vi "Energy(B)INIT.vi"(7 "B [T] in":dbl=1.0, 10 "calib(pixel) out in":T7, 11 "Cam in":T1) -> (2 "calib(pixel) out out":T7, 3 "Cam out 2":T1)   [LabVIEW 2013]
uses:
  calibPixel.ctl
  CamSettingSUB_TypDEf.ctl
  MagAnalysis_Online_Bella/SubVis/CamAndObj_TypDEf.ctl
  shared/OnOffTypeDef.ctl
  userROI.ctl
  shared/numericVariable_TypeDef.ctl
  CamRoiTypDef.ctl
  BaseDriver/BaseDriver.lvclass
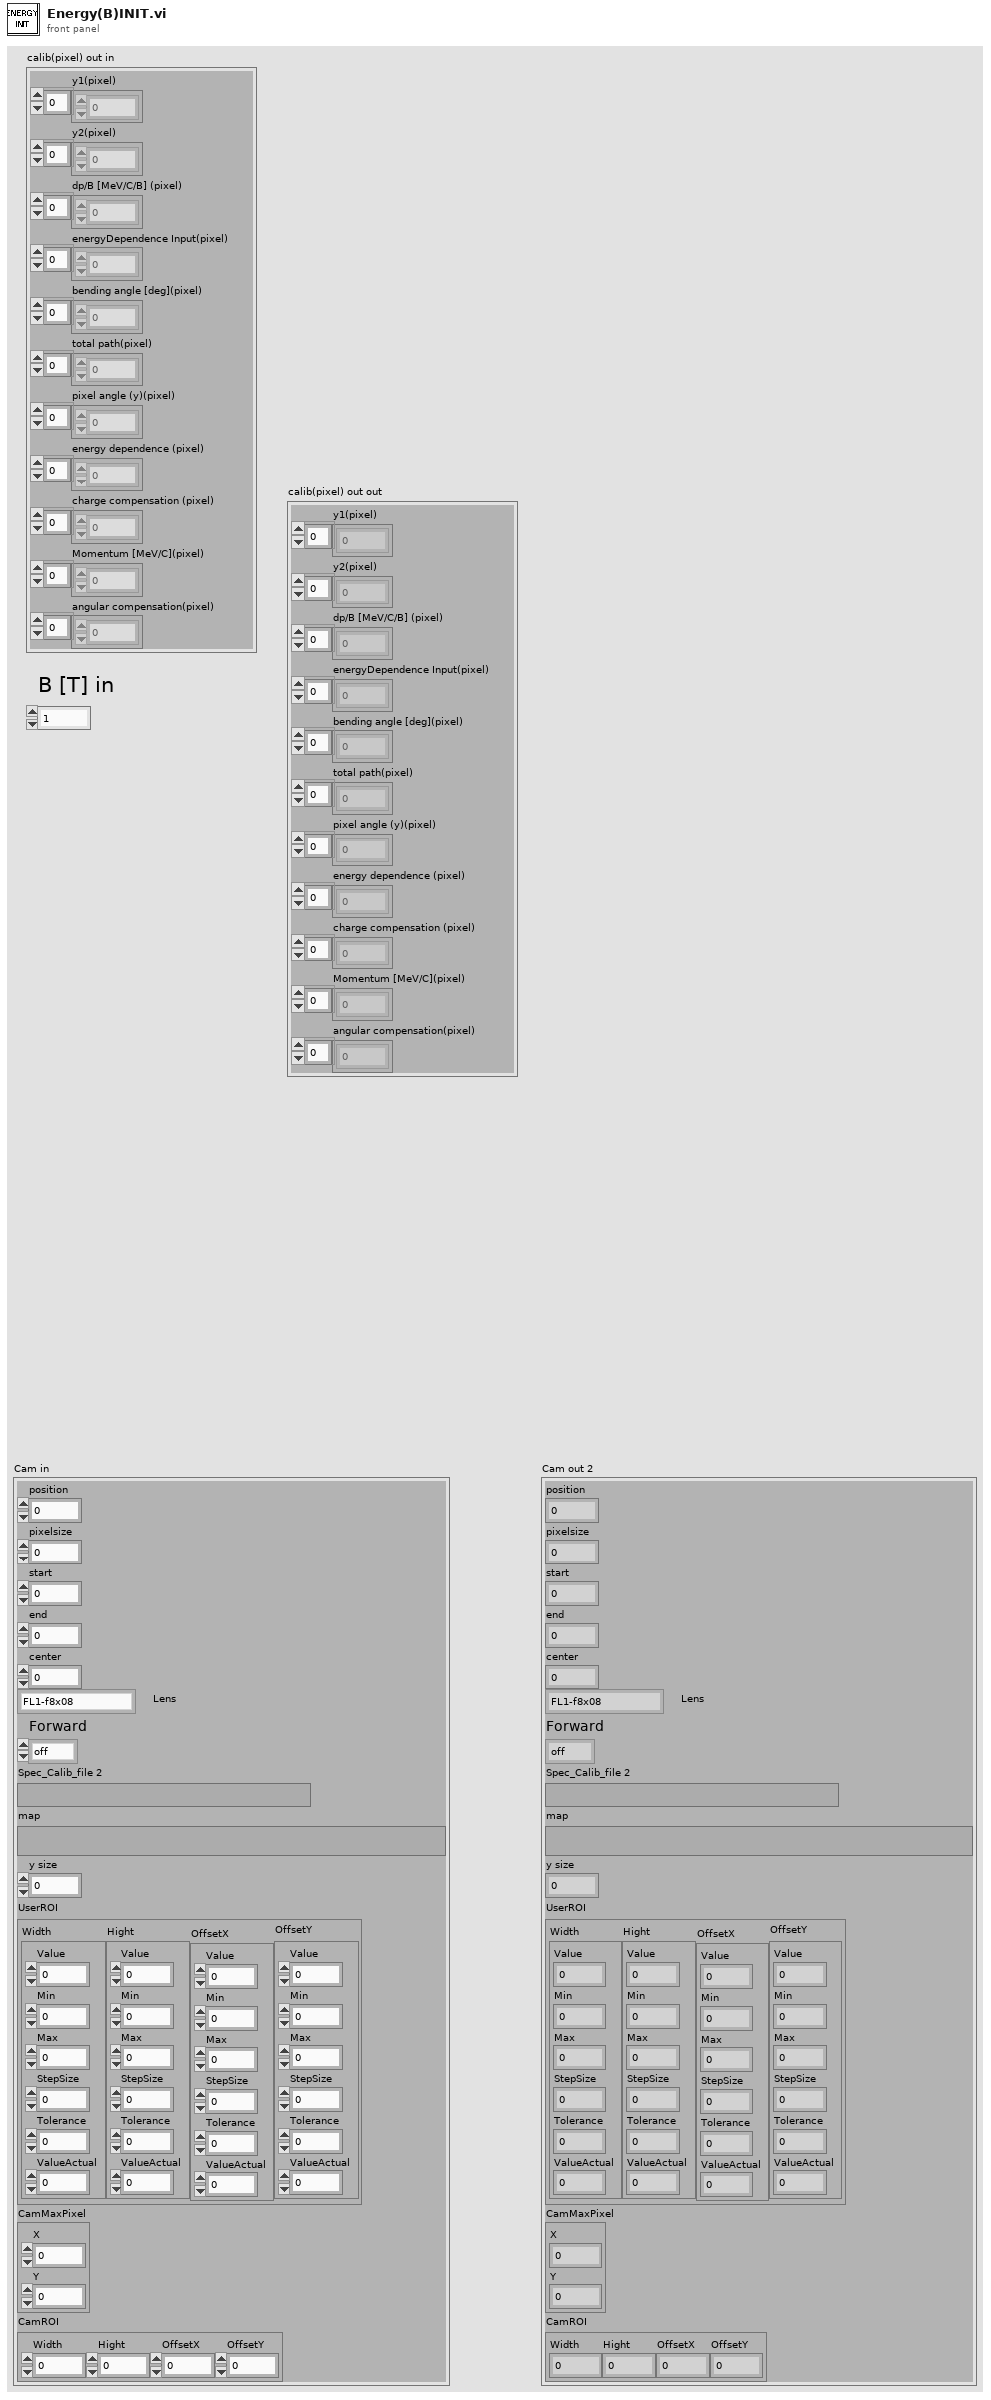
[diagram p1: front panel]
types:
  T1 = typedef "CamSettingSUB_TypDEf.ctl" = cluster{"position":dbl, "pixelsize":dbl, "start":dbl, "end":dbl, "center":dbl, "Lens":T2, "Forward":T3, "Spec_Calib_file 2":path, "map":path, "y size":i32, "UserROI":T4, "CamMaxPixel":cluster{"X":i32, "Y":i32}, "CamROI":T6}
  T2 = typedef "CamAndObj_TypDEf.ctl" = enum16{"FL1-f8x08", "FL1-f8x06", "FL1-f8", "ch300-f50", "FL2G-f8", "FL3M14-f8", "FL3M14-f8x08", "FL3M14-f8x08(2x2)"}
  T3 = typedef "OnOffTypeDef.ctl" = enum16{"off", "on"}
  T4 = typedef "userROI.ctl" = cluster{"Width":T5, "Hight":T5, "OffsetX":T5, "OffsetY":T5}
  T5 = typedef "BaseDriver.lvclass/numericVariable_TypeDef.ctl" = cluster{"Value":dbl, "Min":dbl, "Max":dbl, "StepSize":dbl, "Tolerance":dbl, "ValueActual":dbl}
  T6 = typedef "CamRoiTypDef.ctl" = cluster{"Width":dbl, "Hight":dbl, "OffsetX":dbl, "OffsetY":dbl}
  T7 = typedef "calibPixel.ctl" = cluster{"y1(pixel)":dbl[], "y2(pixel)":dbl[], "dp/B [MeV/C/B] (pixel)":dbl[], "energyDependence Input(pixel)":dbl[], "bending angle [deg](pixel)":dbl[], "total path(pixel)":dbl[], "pixel angle (y)(pixel)":dbl[], "energy dependence (pixel)":dbl[], "charge compensation (pixel)":dbl[], "Momentum [MeV/C](pixel)":dbl[], "angular compensation(pixel)":dbl[]}
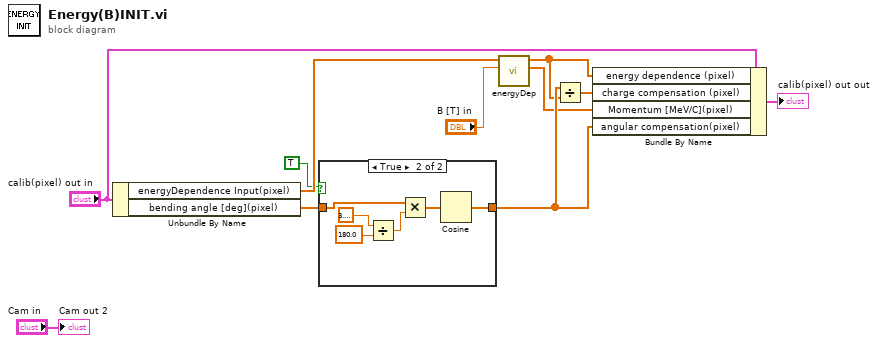
[diagram p0: block diagram]
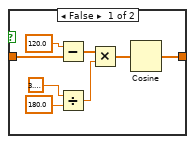
[diagram p2: hidden frame]
diagram:
  n1 = Unbundle By Name("calib(pixel) out in") -> ("energyDependence Input(pixel)"=w10:dbl[], "bending angle [deg](pixel)"=w8:dbl[])
  n2 = case shown="True" TRUE {
    tunnel: w8 -> [w15 w22]
    tunnel: [w12 w20] -> w7
    frame False {
      n3 = Subtract(x=120.0 ("y"), y=w15) -> (x-y=w14:dbl[])
      n4 = Divide(x=3.141592653589793, y=180.0) -> (x/y=w17:dbl)
      n5 = Multiply(x=w14, y=w17) -> (x*y=w13:dbl[])
      n6 = Cosine(x=w13) -> (cos(x)=w12:dbl[])
    }
    frame True {
      n7 = Divide(x=3.141592653589793, y=180.0) -> (x/y=w23:dbl)
      n8 = Multiply(x=w22, y=w23) -> (x*y=w21:dbl[])
      n9 = Cosine(x=w21) -> (cos(x)=w20:dbl[])
    }
  }
  n10 = call "energyDep.vi"("B [T]"="B [T] in", "energy Dep in"=w10) -> ("Momentum [MeV/C]"=w1:dbl[], "energy dependence"=w5:dbl[])  [unwired: 8 in]
  n11 = Divide(x=w7, y=w5) -> (x/y=w6:dbl[])
  n12 = Bundle By Name(cluster="calib(pixel) out in", "energy dependence (pixel)"=w5, "charge compensation (pixel)"=w6, "Momentum [MeV/C](pixel)"=w1, "angular compensation(pixel)"=w7) -> (→"calib(pixel) out out":T7)
  "Cam out 2" <- "Cam in"
